vi "Client watchdog.vi"() -> ()   [LabVIEW 2016]
panel:
  in  "client watchdog":dbl
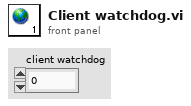
[diagram p1: front panel]
diagram:
